vi "Timing Loop.vi"() -> ()   [LabVIEW 2020]
panel:
  out "millisecond timer value":u32
  out "Output":string
  in  "stop":bool
  out "Elapsed Time (s)":dbl
  out "Random Number":dbl
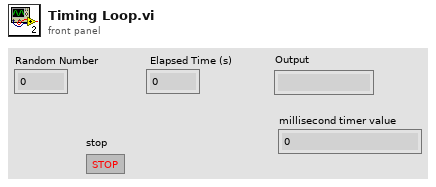
[diagram p1: front panel]
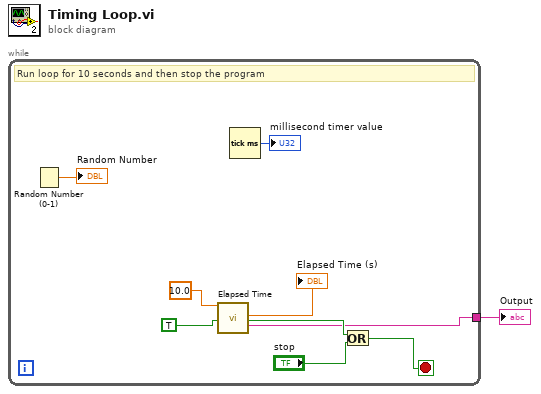
[diagram p0: block diagram]
diagram:
  n1 = while {
    tunnel: [w3] -> w1
    stop <- w6 stop-if-true
    # "Run loop for 10 seconds and then stop the program"
    n2 = Random Number (0-1)() -> (number: 0 to 1=→"Random Number":dbl)
    n3 = call "Elapsed Time"("Time Target (s)"=10.0, "Auto Reset"=TRUE ("Reset")) -> ("Elapsed Time (s)"=→"Elapsed Time (s)":dbl, "Time has Elapsed"=w7:bool, "Elapsed Time Text"=w3:string)  [unwired: 10 in, 5 out]
    n4 = Tick Count (ms)() -> (millisecond timer value=→"millisecond timer value":u32)
    n5 = Or(x=w7, y="stop") -> (x .or. y?=w6:bool)
  }
  "Output" <- w1
